vi "Open Sequence File.vi"(8 "error in (no error)":errorcluster, 10 "Load Options (Default)":T1={"Use Search Dirs? (T)"=TRUE, "Conflict as Error? (T)"=TRUE, "Check Station Model? (F)"=FALSE, "Preload Modules? (T)"=TRUE, "Skip Load Callback? (F)"=FALSE, "Reload if Loaded? (F)"=FALSE}, 11 "Path":path) -> (0 "error out":errorcluster, 3 "Session Handle out":T2)   [LabVIEW 2020, in "TSS.lvlib" / "SequenceFile.lvclass"]
uses:
  SequenceFile.lvclass
  Typedefs/Session Handle.ctl
  Data Types/File Load Options.ctl
  Engine/Engine.lvclass
  TSS.lvlib
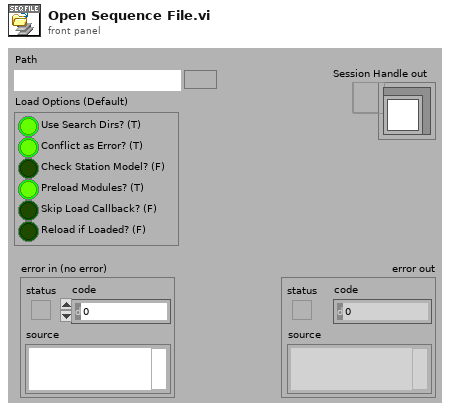
[diagram p1: front panel]
types:
  T1 = typedef "TSS.lvlib/File Load Options.ctl" = cluster{"Use Search Dirs? (T)":bool, "Conflict as Error? (T)":bool, "Check Station Model? (F)":bool, "Preload Modules? (T)":bool, "Skip Load Callback? (F)":bool, "Reload if Loaded? (F)":bool}
  T2 = typedef "TSS.lvlib/SequenceFile.lvclass/Session Handle.ctl" = refnum<data-value>
  T3 = typedef "TSS.lvlib/Engine.lvclass/Session Handle.ctl" = refnum<data-value>
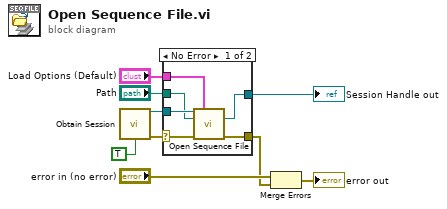
[diagram p0: block diagram]
diagram:
  n1 = call "Obtain Session.vi"("Error to Create? (F)"=TRUE) -> ("Session Handle"=w7:T3, "error out"=w5:errorcluster)  [unwired: 12 in, 1 out]
  n2 = case shown="No Error" w5 {
    selector: w5 -> [w13 w16]
    tunnel: w7 -> [w15 _]
    tunnel: "Load Options (Default)" -> [w14 _]
    tunnel: "Path" -> [w12 _]
    tunnel: [w10 w16] -> w1
    tunnel: [w11 _] -> w3
    frame No Error {
      n3 = call "Open Sequence File.vi"("Engine in"=w15, "Load Options (Default)"=w14, "File Path"=w12, "error in (no error)"=w13) -> ("SequenceFile"=w11:T2, "error out"=w10:errorcluster)  [unwired: 9 in, 1 out]
    }
    frame Error {
    }
  }
  "Session Handle out" <- w3
  n4 = Merge Errors("error in (no error)", w1) -> (→"error out":errorcluster)
